vi "ProcNoticeStr.vi"(11 "Notice Str":string) -> (0 "Msg":string, 1 "Notice ID":T1=enum."OTHERS", 2 "CAN node ID":i32, 3 "Device Index":i32)   [LabVIEW 2016, in "UISimCanFunc_wrapper.lvlib"]
uses:
  <userlib>/UISimCanFunc_wrapper/UISimCanFunc_wrapper.lvlib
  <userlib>/UISimCanFunc_wrapper/ctl/Notice ID.ctl
panel:
  out "错误输出":errorcluster
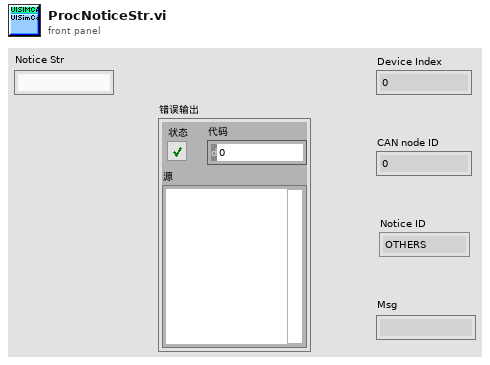
[diagram p1: front panel]
types:
  T1 = typedef "UISimCanFunc_wrapper.lvlib/Notice ID.ctl" = enum16{"S1 FALLING", "S1 RISING", "S2 FALLING", "S2 RISING", "S3 FALLING", "S3 RISING", "P4 DOUT LOW", "P4 DOUT HIGH", "MOVE DONE (OPEN LOOP)", "MOVE DONE (CLOSED LOOP)", "ORIGIN ARRIVED", "STALL NOTIFY", "MOVING", "STANDBY", "SET_TARGET_POS", "OTHERS"}
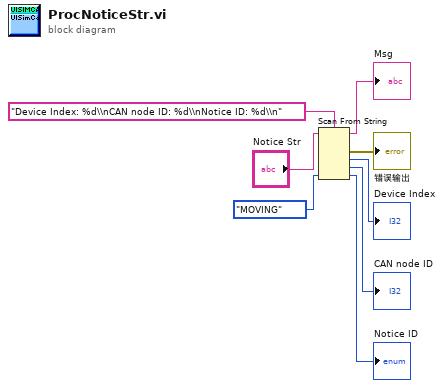
[diagram p0: block diagram]
diagram:
  n1 = Scan From String(format string="Device Index: %d\\nCAN node ID: %d\\nNotice ID: %d\\n", input string="Notice Str", default 3=Notice_ID."MOVING" ("Notice ID 2")) -> (remaining string=→"Msg":string, error out=→"错误输出":errorcluster, output 1=→"Device Index":i32, output 2=→"CAN node ID":i32, output 3=→"Notice ID":T1)  [unwired: 4 in, 1 out]
